vi "Bool Write.vi"(5 "Data Block #":u16, 6 "Bit Offset":u8, 7 "Memory Area":T1, 8 "error in (no error)":errorcluster, 9 "Value":bool, 10 "Start Address":u32, 11 "S7 in":refnum<class "S7NetCom.lvclass">) -> (0 "error out":errorcluster, 3 "S7 out":refnum<class "S7NetCom.lvclass">)   [LabVIEW 2019]
uses:
  <vilib>/Hampel Software Engineering/S7NetCom/Source/S7NetCom.lvclass
  <vilib>/Hampel Software Engineering/S7NetCom/Source/Controls/S7_Memory_Area.ctl
  c84c1ecc-4528-48d3-b92b-584e35eac2f6.vi
  <vilib>/Hampel Software Engineering/S7NetCom/Source/API/Write Data - Boolean (Scalar).vi
  <vilib>/Hampel Software Engineering/S7NetCom/Source/API/Read Data - Boolean (Scalar).vi
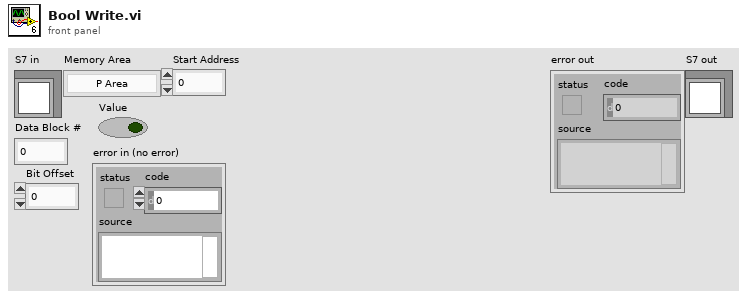
[diagram p1: front panel]
types:
  T1 = typedef "S7NetCom.lvlib/S7NetCom.lvclass/S7_Memory_Area.ctl" = enum8{"P Area", "I Area", "O Area", "M Area", "DB Area", "Counter", "Timer"}
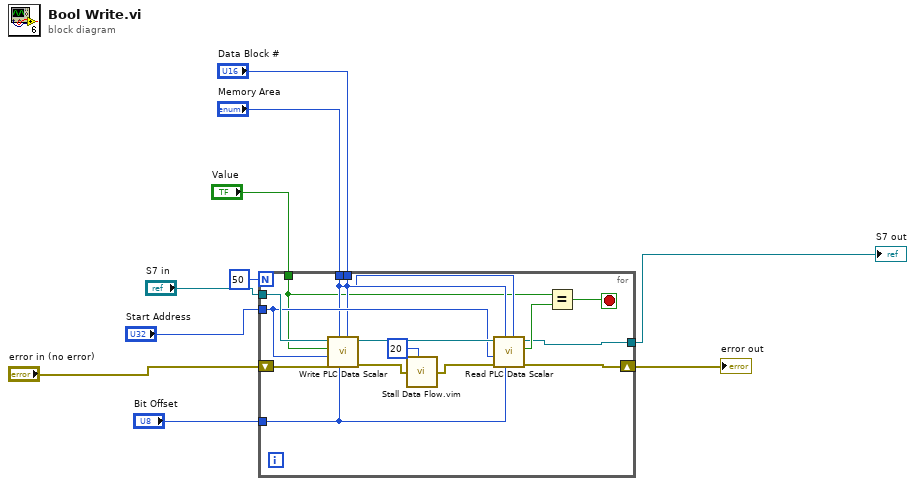
[diagram p0: block diagram]
diagram:
  n1 = for {
    N: 50 -> [_]
    tunnel: "Start Address" -> [w22]
    tunnel: "Memory Area" -> [w21]
    tunnel: "Data Block #" -> [w20]
    tunnel: "Value" -> [w18]
    shift-right: [w17] -> w4
    shift-left: "error in (no error)" -> [w24]
    tunnel: "S7 in" -> [w25]
    tunnel: [w16] -> w3
    tunnel: "Bit Offset" -> [w11]
    stop <- w12 stop-if-true
    n2 = call-poly <vilib>:"Write PLC Data Scalar.vi"("Data Block #"=w20, "Bit Offset"=w11, "Memory Area"=w21, "error in (no error)"=w24, "Start Address"=w22, "Value"=w18, "S7 in"=w25) -> ("error out"=w15:errorcluster, "S7 out"=w23:refnum<class "S7NetCom.lvclass">)  [unwired: 3 in]
    n3 = call "Stall Data Flow.vim"("value in"=w15, "milliseconds to wait"=u32 20) -> ("value out"=w14:errorcluster)  [unwired: 1 out]
    n4 = call-poly <vilib>:"Read PLC Data Scalar.vi"("Data Block #"=w20, "Bit Offset"=w11, "Memory Area"=w21, "error in (no error)"=w14, "Start Address"=w22, "S7 in"=w23) -> ("error out"=w17:errorcluster, "Boolean Value"=w19:bool, "S7 out"=w16:refnum<class "S7NetCom.lvclass">)  [unwired: 3 in]
    n5 = Equal?(x=w18, y=w19) -> (x = y?=w12:bool)
  }
  "error out" <- w4
  "S7 out" <- w3
